vi "Client_bob.vi"   [LabVIEW 2013]
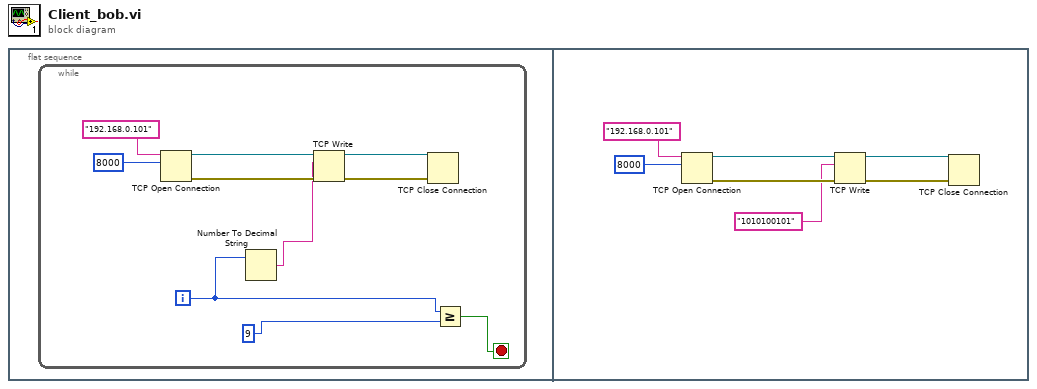
[diagram p0: block diagram]
diagram:
  n1 = flat-sequence {
    frame #0 {
      n2 = while {
        i -> [w2]
        stop <- w3 stop-if-true
        n3 = TCP Open Connection(address="192.168.0.101", remote port or service name=u16 8000) -> (connection ID=w8:refnum<k5>, error out=w5:errorcluster)  [unwired: 3 in]
        n4 = Number To Decimal String(number=w2) -> (decimal integer string=w1:string)  [unwired: 1 in]
        n5 = TCP Write(connection ID=w8, data in=w1, error in (no error)=w5) -> (connection ID out=w6:refnum<k5>, error out=w7:errorcluster)  [unwired: 1 in, 1 out]
        n6 = TCP Close Connection(connection ID=w6, error in (no error)=w7) -> ()  [unwired: 1 in, 2 out]
        n7 = Greater Or Equal?(x=w2, y=9) -> (x >= y?=w3:bool)
      }
    }
    frame #1 {
      n8 = TCP Open Connection(address="192.168.0.101", remote port or service name=u16 8000) -> (connection ID=w13:refnum<k5>, error out=w17:errorcluster)  [unwired: 3 in]
      n9 = TCP Write(connection ID=w13, data in="1010100101", error in (no error)=w17) -> (connection ID out=w16:refnum<k5>, error out=w15:errorcluster)  [unwired: 1 in, 1 out]
      n10 = TCP Close Connection(connection ID=w16, error in (no error)=w15) -> ()  [unwired: 1 in, 2 out]
    }
  }
